vi "Read CPU Temp.vi"(8 "error in (no error)":errorcluster) -> (0 "error out":errorcluster, 2 "Array":dbl[](array[numeric]))   [LabVIEW 2020]
uses:
  C:/Users/Josh/Desktop/code/sandbox/ni/read_temp/OpenHardwareMonitorLib.dll
  OpenHardwareMonitorLib.dll
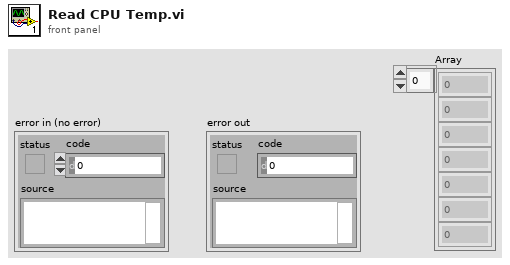
[diagram p1: front panel]
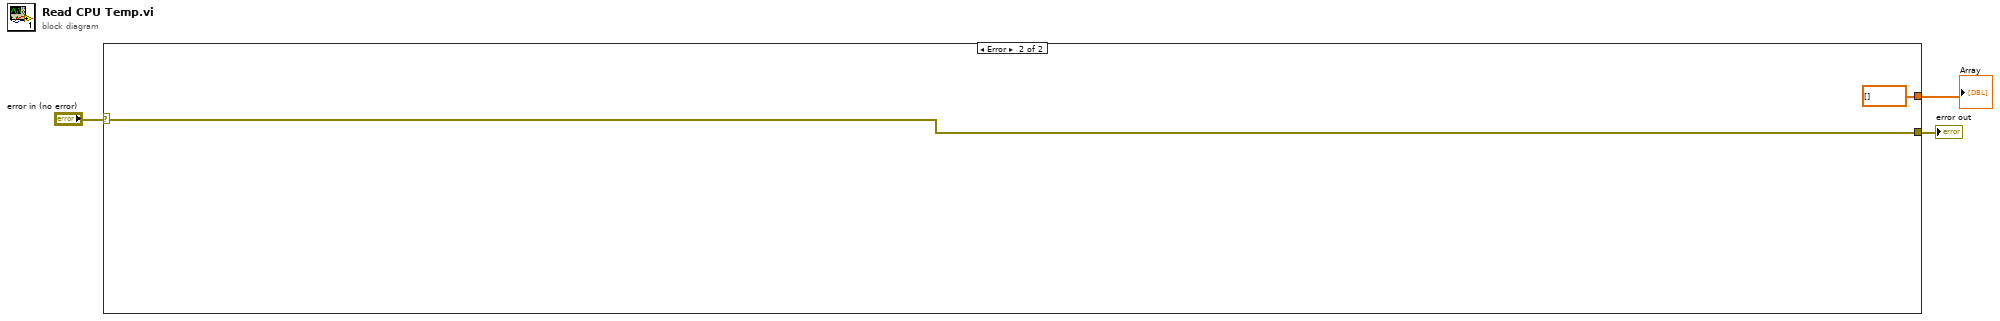
[diagram p0: block diagram]
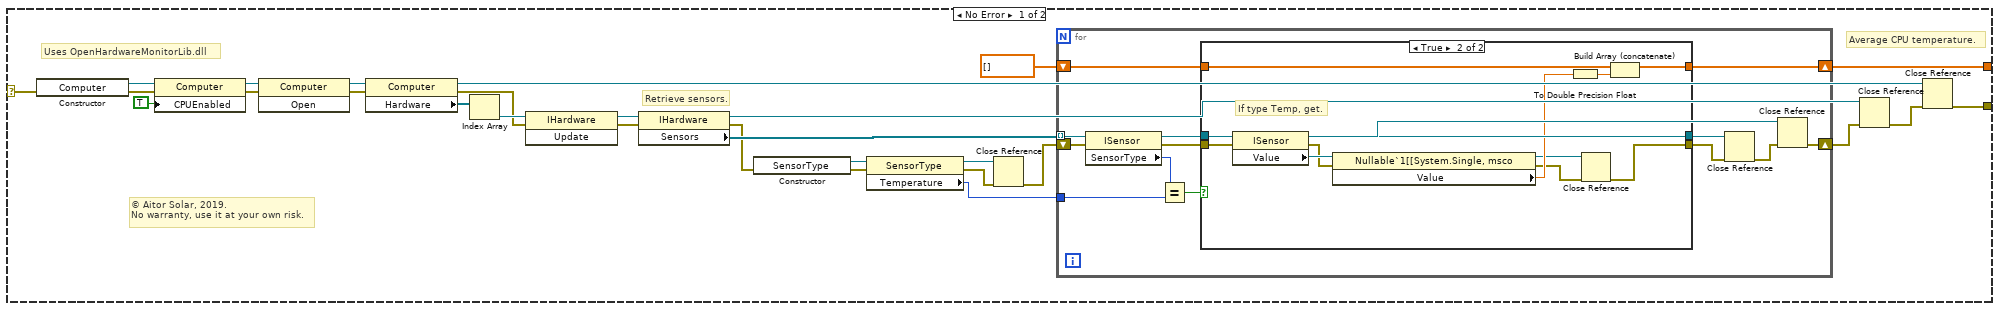
[diagram p2: hidden frame]
diagram:
  n1 = case shown="Error" "error in (no error)" {
    selector: "error in (no error)" -> [w14 w61]
    tunnel: [w15 w61] -> w2
    tunnel: [w4 dbl[] []] -> w1
    frame No Error {
      # "© Aitor Solar, 2019.\nNo warranty, use it at your own risk."
      # "Uses OpenHardwareMonitorLib.dll"
      # "Average CPU temperature."
      # "Retrieve sensors."
      n2 = constructor class="Computer"(error in=w14) -> (reference out=w8:refnum<k24>, error out=w13:errorcluster)  [unwired: 2 in, 1 out]
      n3 = property class="Computer"(reference=w8, error in=w13, "CPUEnabled"=TRUE) -> (reference out=w9:refnum<k24>, error out=w12:errorcluster)
      n4 = invoke class="Computer" method="Open"(reference=w9, error in=w12) -> (reference out=w10:refnum<k24>, error out=w11:errorcluster)  [unwired: 1 in, 1 out]
      n5 = property class="Computer"(reference=w10, error in=w11) -> (reference out=w16:refnum<k24>, error out=w26:errorcluster, "Hardware"=w31:refnum<k24>[])
      n6 = Index Array(array=w31) -> (element=w28:refnum<k24>)  [unwired: 1 in]
      n7 = invoke class="IHardware" method="Update"(reference=w28, error in=w26) -> (reference out=w27:refnum<k24>, error out=w25:errorcluster)  [unwired: 1 in, 1 out]
      n8 = property class="IHardware"(reference=w27, error in=w25) -> (reference out=w18:refnum<k24>, error out=w22:errorcluster, "Sensors"=w29:refnum<k24>[])
      n9 = constructor class="SensorType"(error in=w22) -> (reference out=w23:refnum<k24>, error out=w24:errorcluster)  [unwired: 2 in, 1 out]
      n10 = property class="SensorType"(reference=w23, error in=w24) -> (reference out=w19:refnum<k24>, error out=w6:errorcluster, "Temperature"=w21:i32)
      n11 = Close Reference(reference=w19, error in (no error)=w6) -> (error out=w5:errorcluster)
      n12 = for {
        tunnel: w29 -> [w43] mode=indexing
        shift-right: [w35] -> w7
        shift-left: w5 -> [w42]
        tunnel: w21 -> [w40]
        shift-right: [w44] -> w4
        shift-left: dbl[] [] -> [w38]
        n13 = property class="ISensor"(reference=w43, error in=w42) -> (reference out=w32:refnum<k24>, error out=w41:errorcluster, "SensorType"=w33:i32)
        n14 = Equal?(x=w33, y=w40) -> (x = y?=w39:bool)
        n15 = case shown="True" w39 {
          tunnel: [w47 w58] -> w44
          tunnel: w41 -> [w46 w56]
          tunnel: w38 -> [w47 w59]
          tunnel: [w46 w49] -> w37
          tunnel: [w45 w54] -> w36
          tunnel: w32 -> [w45 w55]
          frame False {
          }
          frame True {
            # "If type Temp, get."
            n16 = property class="ISensor"(reference=w55, error in=w56) -> (reference out=w54:refnum<k24>, error out=w48:errorcluster, "Value"=w53:refnum<k24>)
            n17 = property class="Nullable`1[[System.Single, msco"(reference=w53, error in=w48) -> (reference out=w51:refnum<k24>, error out=w50:errorcluster, "Value"=w52:sgl)
            n18 = To Double Precision Float(number=w52) -> (double precision float=w57:dbl)
            n19 = Close Reference(reference=w51, error in (no error)=w50) -> (error out=w49:errorcluster)
            n20 = Build Array (concatenate)(w59, w57) -> (w58:dbl[])
          }
        }
        n21 = Close Reference(reference=w36, error in (no error)=w37) -> (error out=w34:errorcluster)
        n22 = Close Reference(reference=w32, error in (no error)=w34) -> (error out=w35:errorcluster)
      }
      n23 = Close Reference(reference=w18, error in (no error)=w7) -> (error out=w17:errorcluster)
      n24 = Close Reference(reference=w16, error in (no error)=w17) -> (error out=w15:errorcluster)
    }
    frame Error {
    }
  }
  "error out" <- w2
  "Array" <- w1
